vi "Main Info Bar Message AE.vi"(2 "Action":T1, 7 "Message":string) -> (8 "Message Out":string)   [LabVIEW 2016]
uses:
  Display Module TypeDefs/Display Module Standard Action.ctl
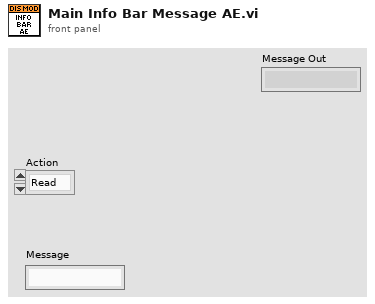
[diagram p1: front panel]
types:
  T1 = typedef "Display Module Standard Action.ctl" = enum16{"Read", "Write"}
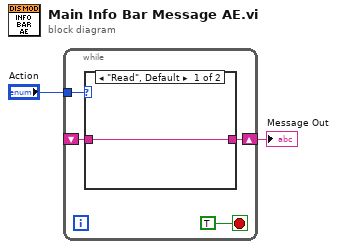
[diagram p0: block diagram]
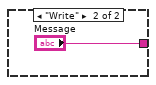
[diagram p2: hidden frame]
diagram:
  n1 = while {
    tunnel: "Action" -> [w5]
    shift-right: [w4] -> w1
    shift-left: _ -> [w3]
    stop <- TRUE stop-if-true
    n2 = case shown="\"Read\", Default" w5 {
      tunnel: [w7 "Message"] -> w4
      tunnel: w3 -> [w7 _]
      frame "Read", Default {
      }
      frame "Write" {
      }
    }
  }
  "Message Out" <- w1
